vi "GetControlOwningPanel.vi"(8 "error in (no error)":errorcluster, 10 "Control Label":string, 11 "CtlLookup In":T1) -> (0 "error out":errorcluster, 1 "Owning VI":refnum<vi>, 2 "Front Panel":refnum<vi>, 3 "CtlLookup Out":T1)   [LabVIEW 2020, in "CtlReferences_API.lvlib"]
doc: "Gets the owning pane and panel of the specified control"
uses:
  CtlReferences_API.lvlib
  CtlReferences/TypeDefs/CtlLookup.ctl
  CtlReferences/CtlReferences.lvclass
  CtlReferences/GetCtlRef.vi
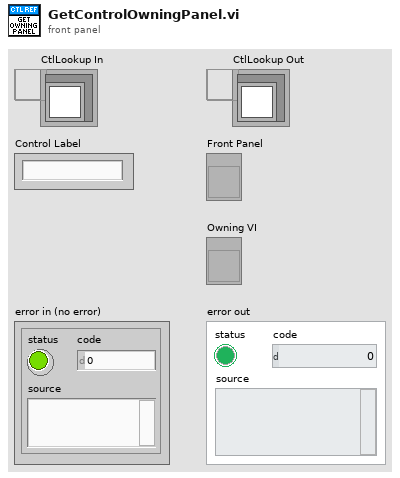
[diagram p1: front panel]
types:
  T1 = typedef "CtlReferences.lvlib/CtlReferences.lvclass/CtlLookup.ctl" = refnum<data-value>
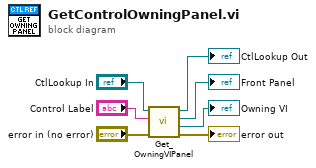
[diagram p0: block diagram]
diagram:
  n1 = call "Get_OwningVIPanel.vi"("error in (no error)"="error in (no error)", "Control Label"="Control Label", "CtlLookup In"="CtlLookup In") -> ("error out"=→"error out":errorcluster, "Owning VI"=→"Owning VI":refnum<vi>, "Front Panel"=→"Front Panel":refnum<vi>, "CtlLookup Out"=→"CtlLookup Out":T1)  [unwired: 5 in]
